vi "Control - Diesel - Air Systems.vi"(0 "Control Inputs":T1={"Engine Speed [RPM]"=0.0, "Engine Status"=enum."STALLED", "Load Control \nMode"=enum."Max Speed Governor", "dt(s)"=0.0, "Number of Cylinders"=0, "Engine Displacement [cc]"=0.0, "StoichAFR"=0.0, "Q.LHV Fuel [kJ/kg]"=0.0, "BattV PSU [V]"=0.0, "12V PSU [V]"=0.0, "5V PSU [V]"=0.0, "Pedal Position [%]"=0.0, "Oil Pressure [kPa]"=0.0, "Oil Temp [C]"=0.0, "Oil Level [%]"=0.0, "Engine Coolant Temp (ECT) [C]"=0.0, "Engine Coolant Pressure [kPa]"=0.0, "Rail Pressure [bar]"=0.0, "Fuel Pressure [kPa]"=0.0, "Fuel Temp [C]"=0.0, "Vacuum Pressure [kPa]"=0.0, "Throttle Position [%]"=0.0, "Cam1 Advance [CAD]"=0.0, "Cam2 Advance [CAD]"=0.0, "Cam3 Advance [CAD]"=0.0, "Cam4 Advance [CAD]"=0.0, "CA50 Control Output [CAD]"=[], "CA50 Control Output Valid"=[], "Intake Air Temp (IAT) [C]"=0.0, "Barometric Air Pressure [kPa]"=0.0, "Intake Air Rel. Humidity [%]"=0.0, "Mass Air Flow (MAF) [kg/hr]"=0.0, "Turbo Inlet Air Pressure [kPa]"=0.0, "Turbo Inlet Air Temp [C]"=0.0, "Turbo Outlet Air Pressure [kPa]"=0.0, "Turbo Outlet Air Temp [C]"=0.0, "CAC Outlet Pressure [kPa]"=0.0, "CAC Outlet Temp [C]"=0.0, "Intake Manifold Pressure (MAP) [kPa]"=0.0, "Intake Manifold Temp (MAT) [C]"=0.0, "Exhaust Manifold Pressure [kPa]"=0.0, "Exhaust Manifold Temp [C]"=0.0, "HighP EGR Cooler Outlet Pressure [kPa]"=0.0, "HighP EGR Cooler Outlet Temp [C]"=0.0, "HighP EGR Differential Pressure [kPa]"=0.0, "HighP EGR Valve Position [%]"=0.0, "Turbo Outlet Exhaust Pressure [kPa]"=0.0, "Turbo Outlet Exhaust Temp [C]"=0.0, "VGT Position 1 [%]"=0.0, "VGT Position 2 [%]"=0.0, "Turbo Speed 1 [RPM]"=0.0, "Turbo Speed 2 [RPM]"=0.0, "LowP EGR Differential Pressure [kPa]"=0.0, "LowP EGR Valve Position [%]"=0.0, "UEGO1Lambda"=0.0, "UEGO1_Hot"=FALSE, "UEGO2Lambda"=0.0, "UEGO2_Hot"=FALSE, "Knock Intensity"=[], "Knock"=[]} {"Knock Intensity" format="%.2f"; "CA50 Control Output [CAD]" format="%.2f"; "Exhaust Manifold Temp [C]" format="%#_6f"; "UEGO2Lambda" format="%.2f"; "Intake Manifold Temp (MAT) [C]" format="%#_6f"; "UEGO1Lambda" format="%.2f"}, 1 "MEP Desired [bar]":sgl, 2 "Fuel Desired [mg/cyc] (Fdbk)":sgl) -> (11 "Intake MAP Desired [kPa]":sgl, 13 "Available Air Mass [mg/cyc]":sgl, 14 "Cam1 Advance [CAD]":sgl, 15 "Cam2 Advance [CAD]":sgl, 16 "VGT Position [%Closed]":sgl, 17 "Wastegate Position [%Open]":sgl, 18 "High-Pressure EGR Position [%Open]":sgl, 19 "Low-Pressure EGR Position [%Open]":sgl)   [LabVIEW 2015, in "ECS-RT.lvlib"]
uses:
  ECS-RT.lvlib
  Typedefs/Control Inputs/Control Inputs.ctl
  Typedefs/EPT/Engine Status.ctl
  Typedefs/MISC/Load Control Mode.ctl
  ECS-Shared.lvlib
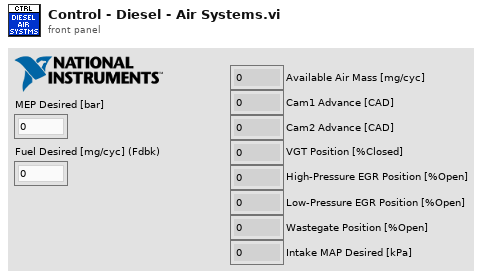
[diagram p1: front panel]
types:
  T1 = typedef "ECS-Shared.lvlib/Control Inputs.ctl" = cluster{"Engine Speed [RPM]":sgl, "Engine Status":T2, "Load Control \nMode":T3, "dt(s)":sgl, "Number of Cylinders":u8, "Engine Displacement [cc]":sgl, "StoichAFR":sgl, "Q.LHV Fuel [kJ/kg]":sgl, "BattV PSU [V]":sgl, "12V PSU [V]":sgl, "5V PSU [V]":sgl, "Pedal Position [%]":sgl, "Oil Pressure [kPa]":sgl, "Oil Temp [C]":sgl, "Oil Level [%]":sgl, "Engine Coolant Temp (ECT) [C]":sgl, "Engine Coolant Pressure [kPa]":sgl, "Rail Pressure [bar]":sgl, "Fuel Pressure [kPa]":sgl, "Fuel Temp [C]":sgl, "Vacuum Pressure [kPa]":sgl, "Throttle Position [%]":sgl, "Cam1 Advance [CAD]":sgl, "Cam2 Advance [CAD]":sgl, "Cam3 Advance [CAD]":sgl, "Cam4 Advance [CAD]":sgl, "CA50 Control Output [CAD]":sgl[], "CA50 Control Output Valid":bool[], "Intake Air Temp (IAT) [C]":sgl, "Barometric Air Pressure [kPa]":sgl, "Intake Air Rel. Humidity [%]":sgl, "Mass Air Flow (MAF) [kg/hr]":sgl, "Turbo Inlet Air Pressure [kPa]":sgl, "Turbo Inlet Air Temp [C]":sgl, "Turbo Outlet Air Pressure [kPa]":sgl, "Turbo Outlet Air Temp [C]":sgl, "CAC Outlet Pressure [kPa]":sgl, "CAC Outlet Temp [C]":sgl, "Intake Manifold Pressure (MAP) [kPa]":sgl, "Intake Manifold Temp (MAT) [C]":sgl, "Exhaust Manifold Pressure [kPa]":sgl, "Exhaust Manifold Temp [C]":sgl, "HighP EGR Cooler Outlet Pressure [kPa]":sgl, "HighP EGR Cooler Outlet Temp [C]":sgl, "HighP EGR Differential Pressure [kPa]":sgl, "HighP EGR Valve Position [%]":sgl, "Turbo Outlet Exhaust Pressure [kPa]":sgl, "Turbo Outlet Exhaust Temp [C]":sgl, "VGT Position 1 [%]":sgl, "VGT Position 2 [%]":sgl, "Turbo Speed 1 [RPM]":sgl, "Turbo Speed 2 [RPM]":sgl, "LowP EGR Differential Pressure [kPa]":sgl, "LowP EGR Valve Position [%]":sgl, "UEGO1Lambda":sgl, "UEGO1_Hot":bool, "UEGO2Lambda":sgl, "UEGO2_Hot":bool, "Knock Intensity":sgl[], "Knock":bool[]}
  T2 = typedef "ECS-Shared.lvlib/Engine Status.ctl" = enum16{"OFF", "STALLED", "CRANKING", "RUNNING", "ACCEL", "DECEL", "SAFE"}
  T3 = typedef "ECS-Shared.lvlib/Load Control Mode.ctl" = enum16{"No Governor", "Min Speed Governor", "Max Speed Governor"}
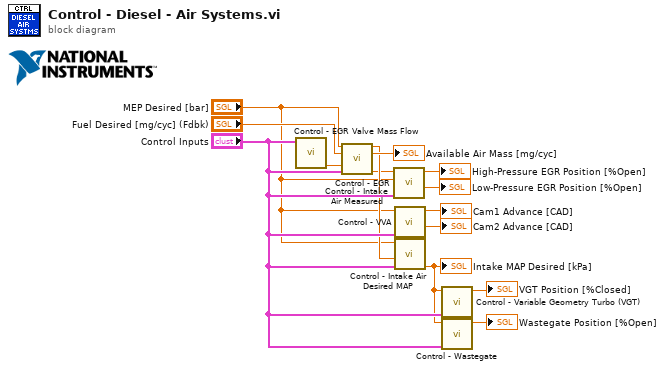
[diagram p0: block diagram]
diagram:
  n1 = call "Control - EGR Valve Mass Flow.vi"("Control Inputs"="Control Inputs") -> ("EGR Mass Flow [kg/hr]"=w7:sgl)  [unwired: 10 in]
  n2 = call "Control - Intake Air Measured.vi"("MEP Desired [bar] (MAF w/ EGR Only)"="MEP Desired [bar]", "Fuel [mg/cyc] (Fdbk)"="Fuel Desired [mg/cyc] (Fdbk)", "Pre-Calculated EGR Mass Flow [kg/hr] (MAP Only)"=w7, "Control Inputs"="Control Inputs") -> ("Volumetric Efficiency [%]"=w3:sgl, "Available Air Mass [mg/cyc]"=→"Available Air Mass [mg/cyc]":sgl, "EGR Mass [mg/cyc]"=w2:sgl)  [unwired: 7 in, 2 out]
  n3 = call "Control - EGR.vi"("Control Inputs"="Control Inputs", "MEP Desired [bar]"="MEP Desired [bar]", "EGR Mass [mg/cyc]"=w2) -> ("Low-Pressure EGR Position [%Open]"=→"Low-Pressure EGR Position [%Open]":sgl, "High-Pressure EGR Position [%Open]"=→"High-Pressure EGR Position [%Open]":sgl)  [unwired: 7 in]
  n4 = call "Control - VVA.vi"("Control Inputs"="Control Inputs", "MEP Desired [bar]"="MEP Desired [bar]") -> ("Cam2 Advance [CAD]"=→"Cam2 Advance [CAD]":sgl, "Cam1 Advance [CAD]"=→"Cam1 Advance [CAD]":sgl)  [unwired: 7 in]
  n5 = call "Control - Intake Air Desired MAP.vi"("Control Inputs"="Control Inputs", "Volumetric Efficiency [%]"=w3, "MEP Desired [bar]"="MEP Desired [bar]") -> ("Intake MAP Desired [kPa]"=w4:sgl)  [unwired: 7 in, 1 out]
  "Intake MAP Desired [kPa]" <- w4
  n6 = call "Control - Variable Geometry Turbo (VGT).vi"("Control Inputs"="Control Inputs", "Intake MAP Desired [kPa]"=w4) -> ("VGT Position [%Open]"=→"VGT Position [%Closed]":sgl)  [unwired: 9 in]
  n7 = call "Control - Wastegate.vi"("Control Inputs"="Control Inputs", "Intake MAP Desired [kPa]"=w4) -> ("Wastegate Position [%Open]"=→"Wastegate Position [%Open]":sgl)  [unwired: 9 in]
